vi "Trigger Conversion.vi"(1 "R2":i32) -> (0 "Array":i32[](array[numeric]))   [LabVIEW 2021]
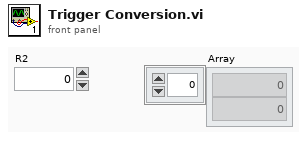
[diagram p1: front panel]
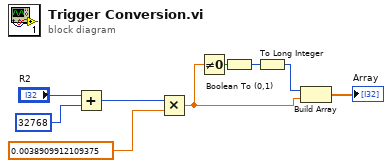
[diagram p0: block diagram]
diagram:
  n1 = Add(x="R2", y=32768) -> (x+y=w4:i32)
  n2 = Multiply(x=w4, y=0.0038909912109375) -> (x*y=w1:dbl)
  n3 = Not Equal To 0?(x=w1) -> (x != 0?=w9:bool)
  n4 = Boolean To (0,1)(Boolean=w9) -> (0, 1=w6:i16)
  n5 = To Long Integer(number=w6) -> (32bit integer=w8:i32)
  n6 = Build Array(w8, w1) -> (→"Array":dbl[])
